vi "getTaskInfo_byName.vi"(10 "TaskName":string, 11 "ActiveTask in":T1(array[cluster])) -> (0 "index":i32, 1 "found?":bool, 2 "TaskInfo":cluster{"TaskName":string, "TaskRef":refnum<vi>}, 3 "ActiveTask out":T1(array[cluster]))   [LabVIEW 2015, in "pdbm_test_system.lvlib"]
uses:
  pdbm_test_system.lvlib
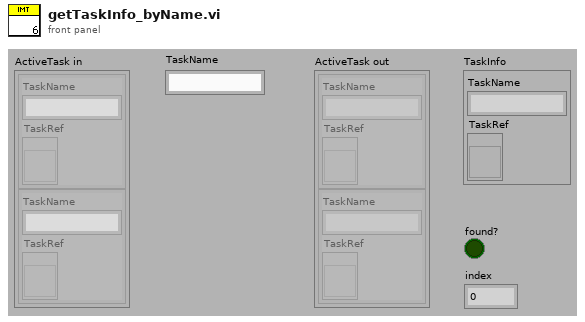
[diagram p1: front panel]
types:
  T1 = cluster{"TaskName":string, "TaskRef":refnum<vi>}[]
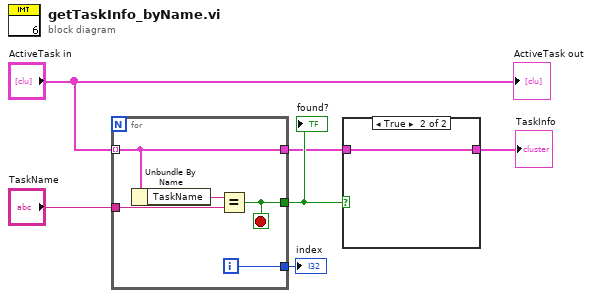
[diagram p0: block diagram]
diagram:
  n1 = for {
    tunnel: "ActiveTask in" -> [w7] mode=indexing
    tunnel: "TaskName" -> [w11]
    tunnel: [w9] -> w4
    tunnel: [w7] -> w3
    tunnel: [w8] -> w2
    i -> [w8]
    stop <- w9 stop-if-true
    n2 = Unbundle By Name(w7) -> ("TaskName"=w10:string)
    n3 = Equal?(x=w10, y=w11) -> (x = y?=w9:bool)
  }
  "found?" <- w4
  "index" <- w2
  n4 = case shown="True" w4 {
    tunnel: w3 -> [_ w12]
    tunnel: [_ w12] -> w1
    frame False {
    }
    frame True {
    }
  }
  "TaskInfo" <- w1
  "ActiveTask out" <- "ActiveTask in"
